vi "New motor Control integrated (old).vi"(2 "wTargetSpeed":dbl(slide) scale=-1.0..1.0, 3 "yTargetSpeed":dbl(slide) scale=-1.0..1.0, 4 "xTargetSpeed":dbl(slide) scale=-1.0..1.0, 5 "Reset Encoders":bool) -> (0 "Speed":T2, 1 "Distance":T1)   [LabVIEW 2018]
panel:
  out "Motor Error":errorcluster
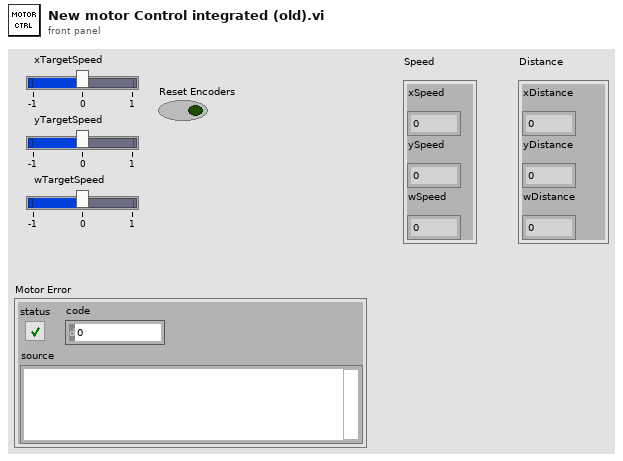
[diagram p1: front panel]
types:
  T1 = cluster{"xDistance":dbl, "yDistance":dbl, "wDistance":dbl}
  T2 = cluster{"xSpeed":dbl, "ySpeed":dbl, "wSpeed":dbl}
  T3 = cluster{"Encoder 0":dbl, "Encoder 1":dbl, "Encoder 2":dbl}
  T4 = cluster{"Distance M0 ":dbl, "Distance M1 ":dbl, "Distance M2 ":dbl}
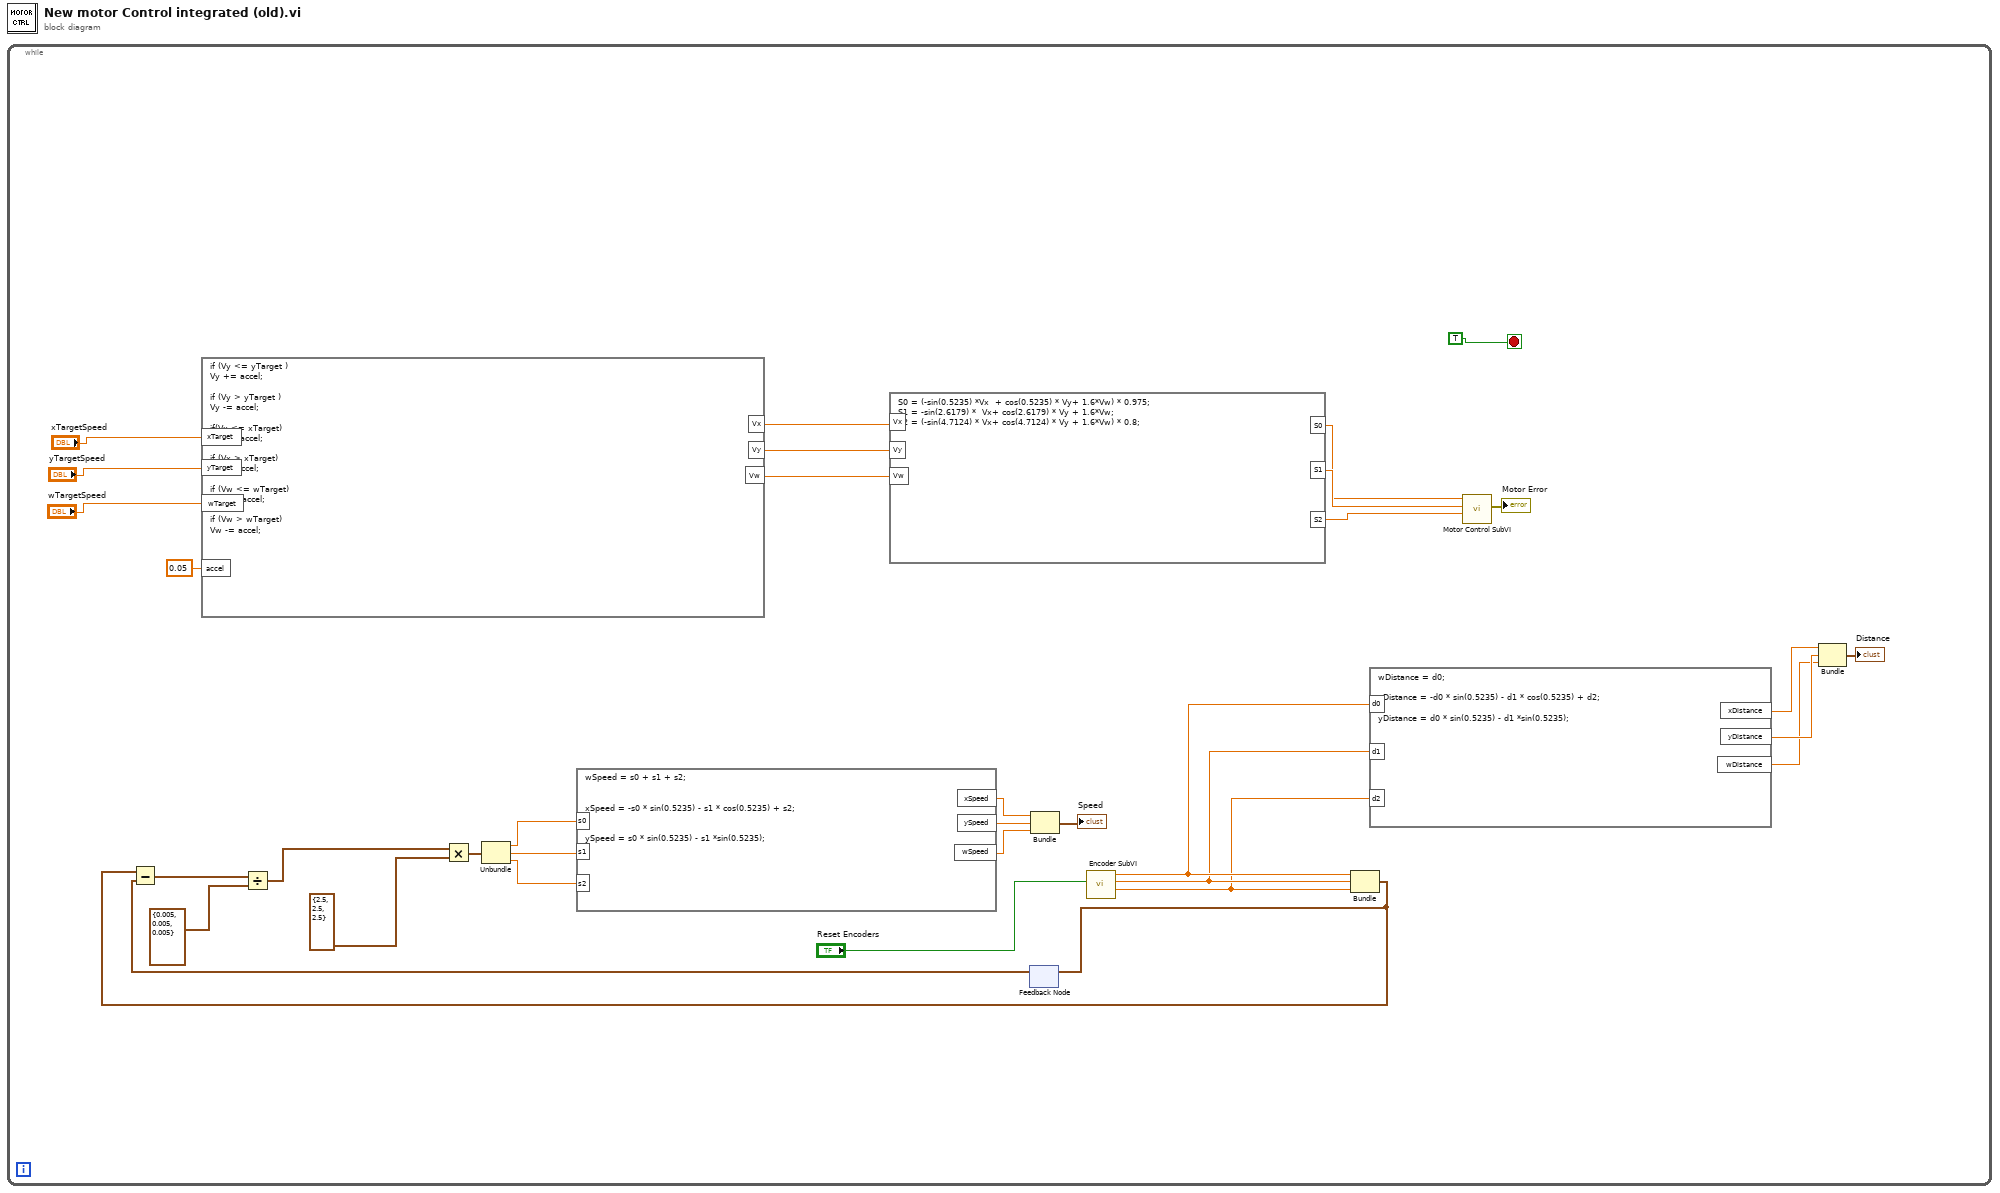
[diagram p0: block diagram]
diagram:
  n1 = while {
    stop <- TRUE ("Boolean") stop-if-true
    n2 = formula code="if (Vy <= yTarget )\nVy += accel;\n\nif (Vy > yTarget )\nVy -= accel;\n\nif(Vx <= xTarget)\nVx += accel;\n\nif (Vx > xTarget)\nVx -= accel;\n\nif (Vw <= wTarget)\nVw += accel;\n\nif (Vw > wTarget)\nVw -= accel;"("xTarget"="xTargetSpeed", "yTarget"="yTargetSpeed", "wTarget"="wTargetSpeed", "accel"=0.05 ("input variable")) -> ("Vy"=w8:dbl, "Vx"=w6:dbl, "Vw"=w7:dbl)
    n3 = formula code="S0 = (-sin(0.5235) *Vx  + cos(0.5235) * Vy+ 1.6*Vw) * 0.975;\nS1 = -sin(2.6179) *  Vx+ cos(2.6179) * Vy + 1.6*Vw;\nS2 = (-sin(4.7124) * Vx+ cos(4.7124) * Vy + 1.6*Vw) * 0.8;"("Vx"=w6, "Vy"=w8, "Vw"=w7) -> ("S0"=w12:dbl, "S1"=w25:dbl, "S2"=w24:dbl)
    n4 = feedback #1() -> (w23:T4)  [unwired: 1 in]
    n5 = call "Encoder SubVI.vi"("Reset Encoders"="Reset Encoders") -> ("Distance M2"=w20:dbl, "Distance M1"=w21:dbl, "Distance M0"=w22:dbl)  [unwired: 7 in, 1 out]
    n6 = Bundle("Distance M0"=w22, "Distance M1"=w21, "Distance M2"=w20) -> (w9:T4)  [unwired: 1 in]
    n7 = Subtract(x=w9, y=w23) -> (x-y=w34:T4)
    n8 = Divide(x=w34, y=T3 {"Encoder 0"=0.005, "Encoder 1"=0.005, "Encoder 2"=0.005}) -> (x/y=w15:cluster{dbl, dbl, dbl})
    n9 = Multiply(x=w15, y=cluster{dbl, dbl, dbl} {2.5, 2.5, 2.5}) -> (x*y=w13:cluster{dbl, dbl, dbl})
    n10 = Unbundle(w13) -> (w11:dbl, w27:dbl, w26:dbl)
    n11 = formula code="wSpeed = s0 + s1 + s2;\n\n\nxSpeed = -s0 * sin(0.5235) - s1 * cos(0.5235) + s2;\n\n\nySpeed = s0 * sin(0.5235) - s1 *sin(0.5235);"("s0"=w11, "s1"=w27, "s2"=w26) -> ("xSpeed"=w31:dbl, "ySpeed"=w32:dbl, "wSpeed"=w30:dbl)
    n12 = feedback-in #1(w9) -> ()
    n13 = Bundle("xSpeed"=w31, "ySpeed"=w32, "wSpeed"=w30) -> (→"Speed":T2)  [unwired: 1 in]
    n14 = formula code="wDistance = d0;\n\nxDistance = -d0 * sin(0.5235) - d1 * cos(0.5235) + d2;\n\nyDistance = d0 * sin(0.5235) - d1 *sin(0.5235);"("d0"=w22, "d1"=w21, "d2"=w20) -> ("xDistance"=w19:dbl, "wDistance"=w17:dbl, "yDistance"=w18:dbl)
    n15 = call "Motor Control SubVI.vi"("Speed M2"=w24, "Speed M1"=w25, "Speed M0"=w12) -> ("Motor Error"=→"Motor Error":errorcluster)  [unwired: 8 in]
    n16 = Bundle("xDistance"=w19, "yDistance"=w18, "wDistance"=w17) -> (→"Distance":T1)  [unwired: 1 in]
  }
